vi "Main.vi"() -> ()   [LabVIEW 2021]
doc: "Use this template to build a simple state machine design pattern. Each state executes code and determines which state to transition to."
uses:
  controls/State.ctl
  controls/Data.ctl
  vmmso/vmmso.lvlib
panel:
  in  "DDS2 Amplitude":dbl=2000.0
  in  "DDS2 Bias":dbl
  in  "DDS2 Freq":dbl=1000.0
  in  "DDS2 Wave Style":u16(ring) items=["Sine", "Square", "Ramp"]
  in  "DDS1 Amplitude":dbl=2000.0
  in  "DDS1 Bias":dbl
  in  "DDS1 Freq":dbl=1000.0
  in  "DDS1 Wave Style":u16(ring) items=["Sine", "Square", "Ramp"]
  out "Is Data Ready？":bool
  out "ReadVoltageData Return":u32
  out "Voltage Wave":dbl[][](graph)
  out "Capture Return":i32
  out "Device is OK?":bool
  out "Support Samples":u32[](array[numeric])
  in  "Exit":bool
  # "DDS1"
  # "DDS2"
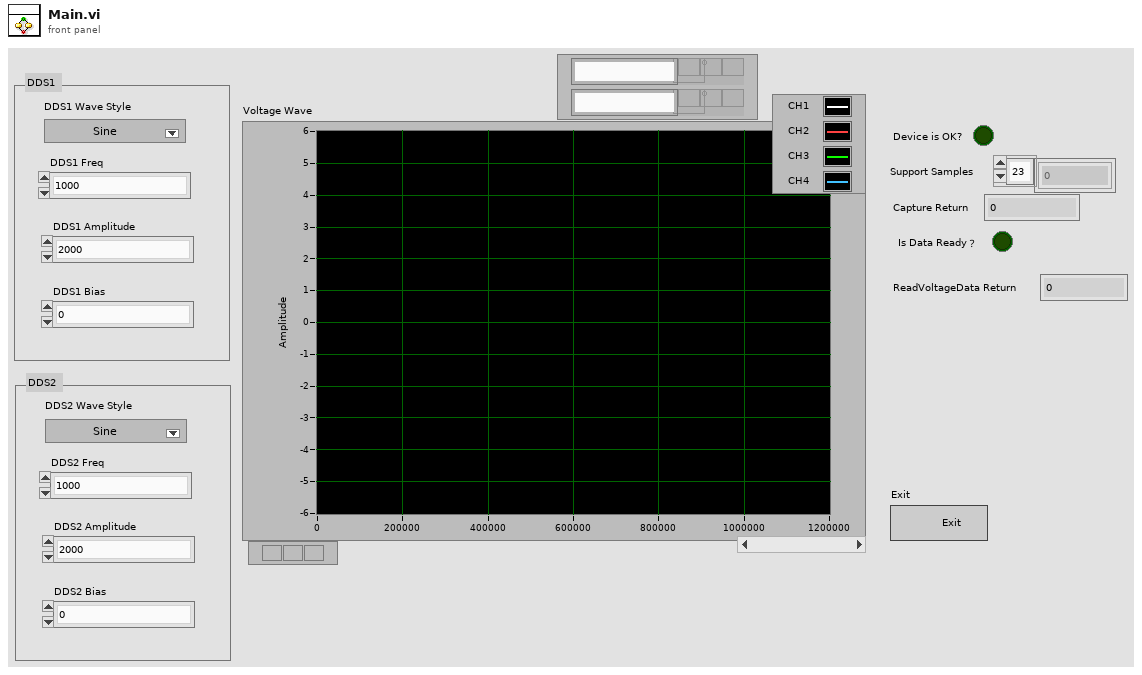
[diagram p1: front panel]
types:
  T1 = typedef "Data.ctl" = cluster{"Boolean <Replace Me>":bool, "String <Replace Me>":string, "Numeric <Replace Me>":dbl}
  T2 = typedef "State.ctl" = enum16{"Initialize", "Wait for UsbIn", "Init Osc and Dds", "Wait for Event", "Capture", "Read Voltage", "Exit"}
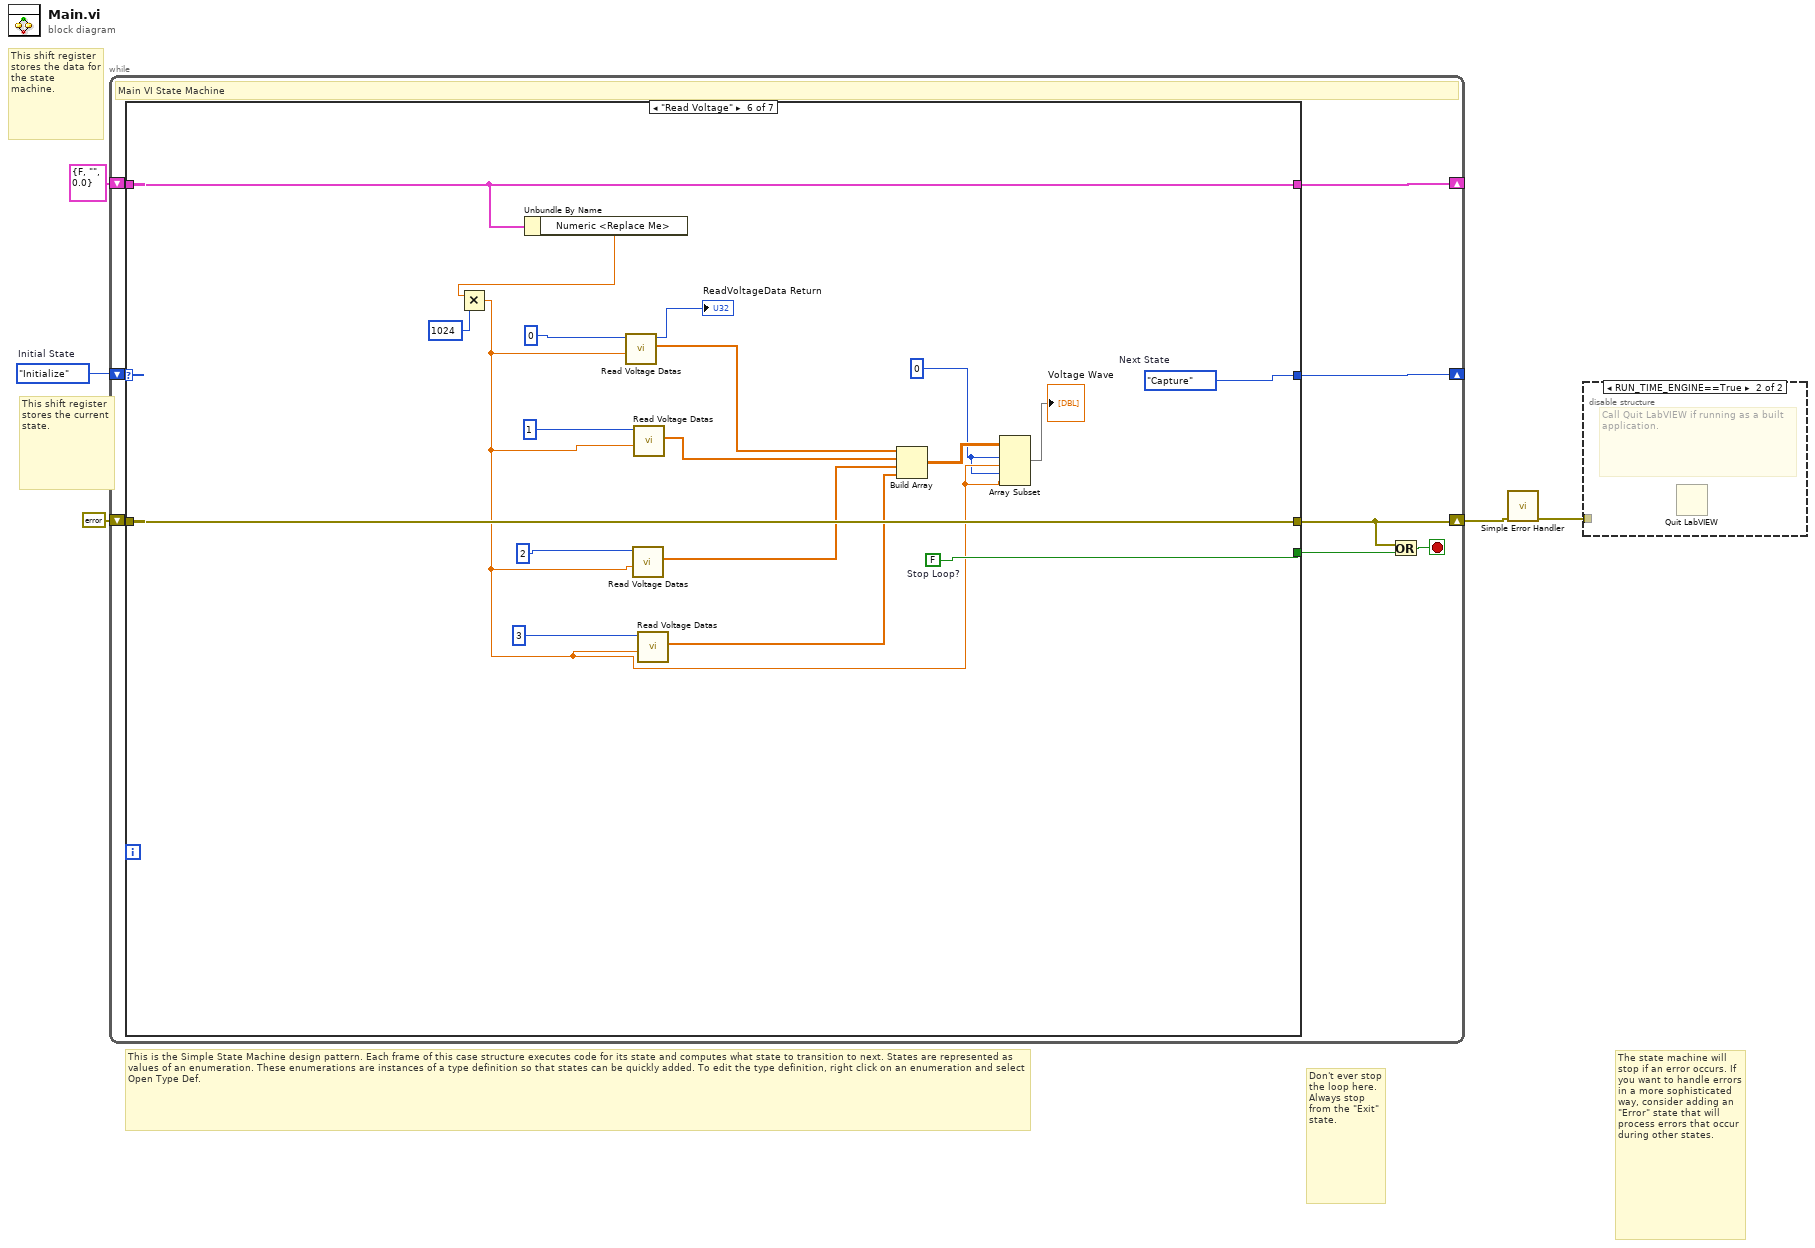
[diagram p0: block diagram]
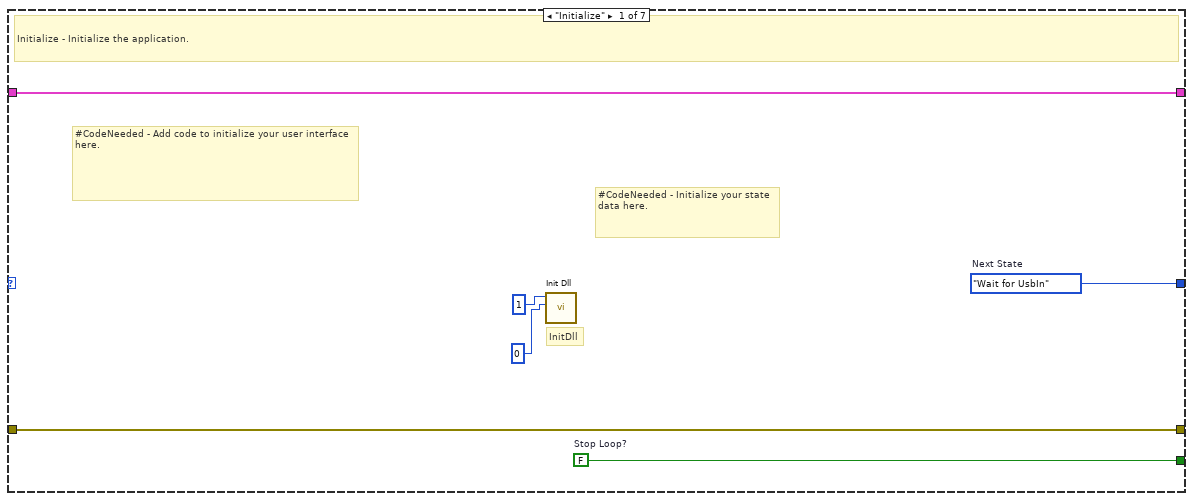
[diagram p3: hidden frame]
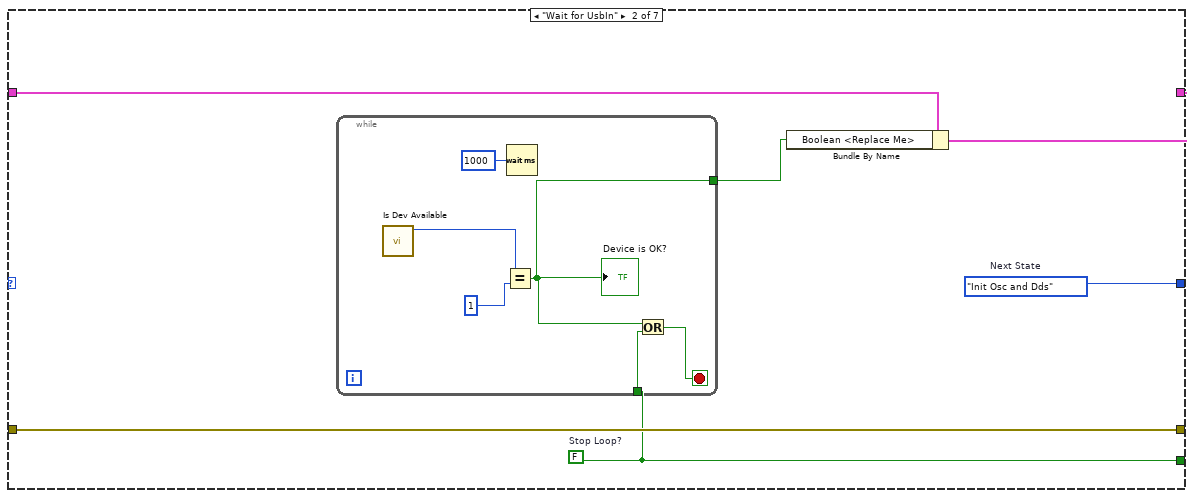
[diagram p4: hidden frame]
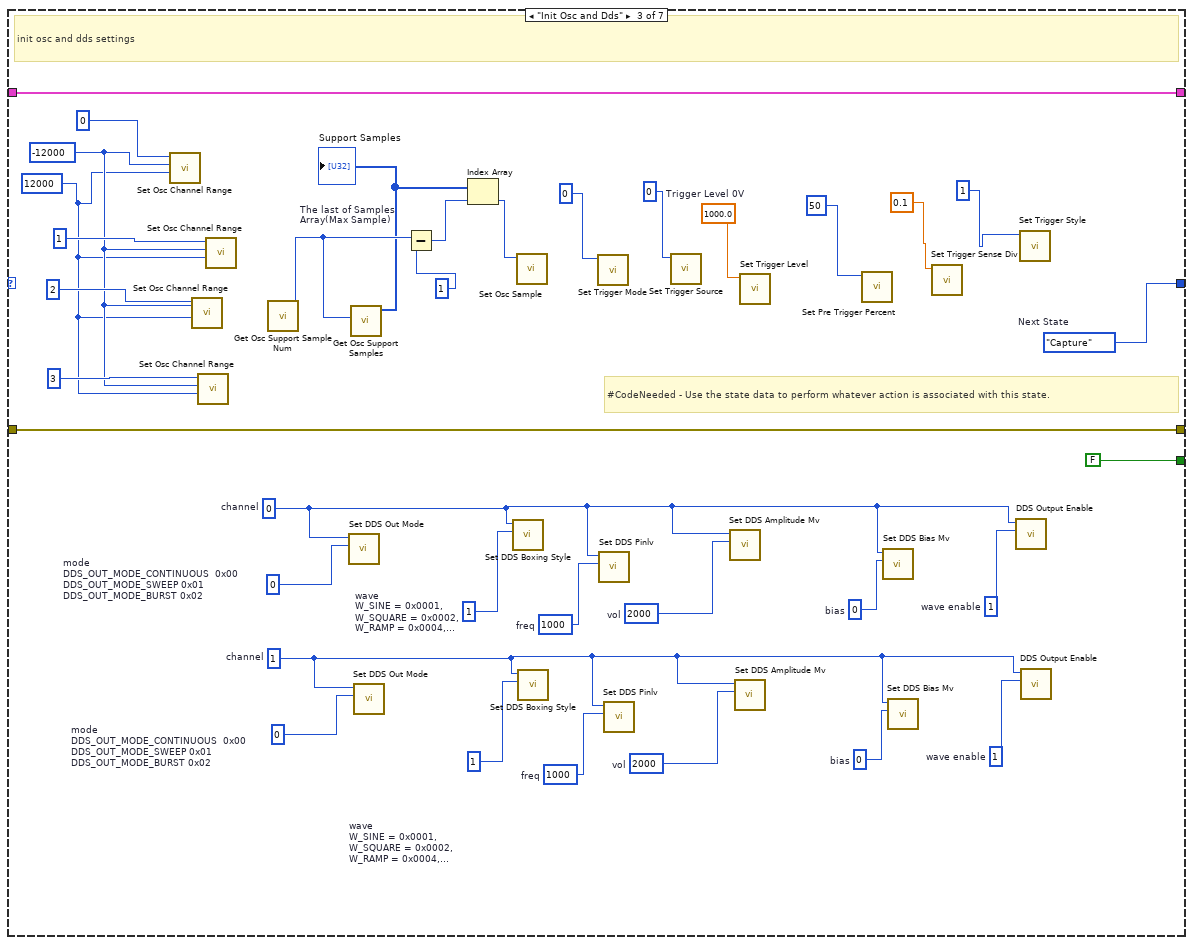
[diagram p5: hidden frame]
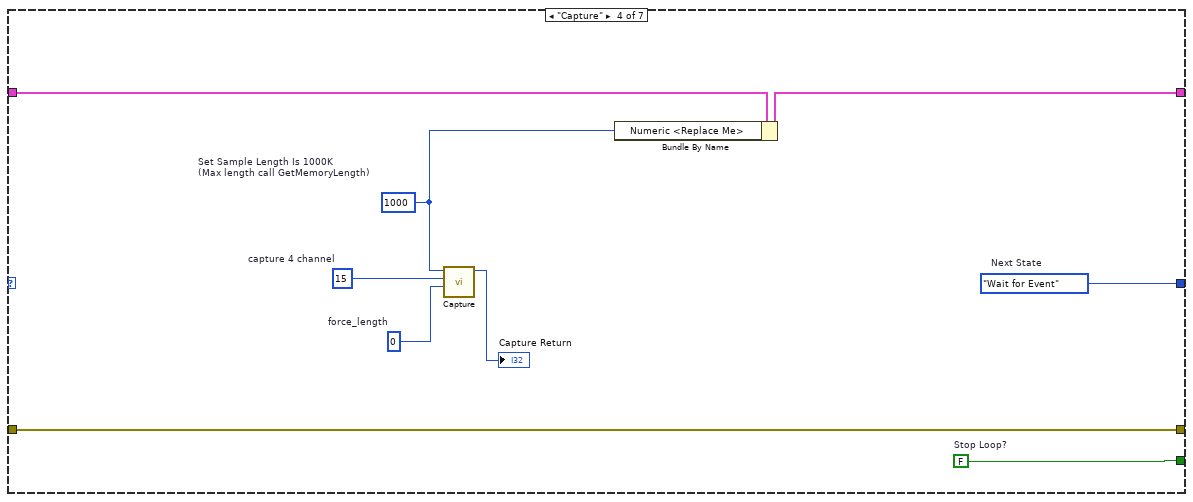
[diagram p6: hidden frame]
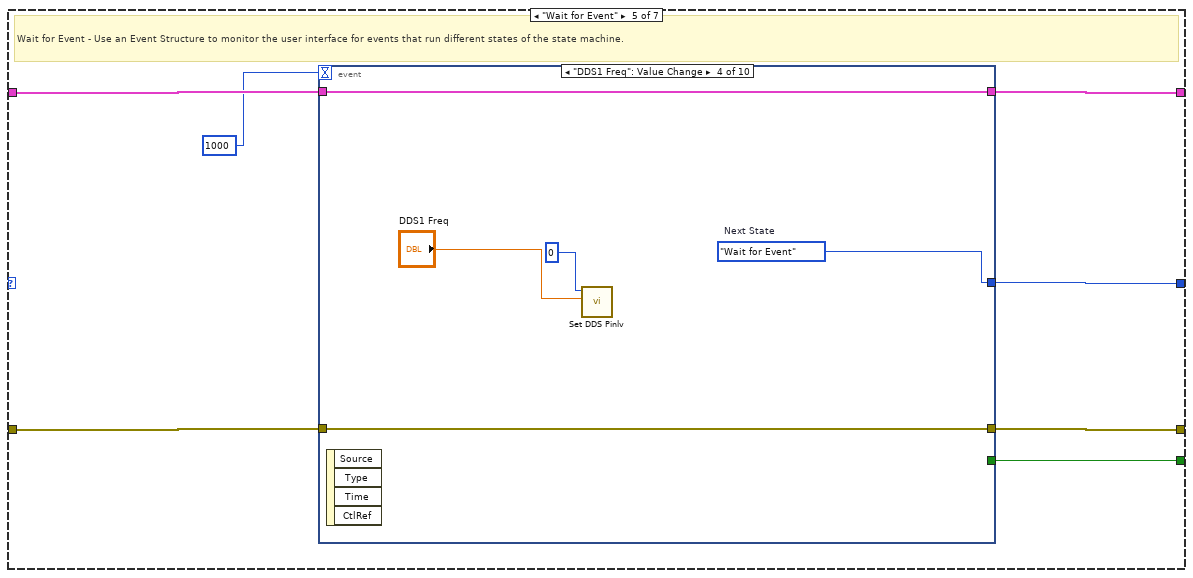
[diagram p7: hidden frame]
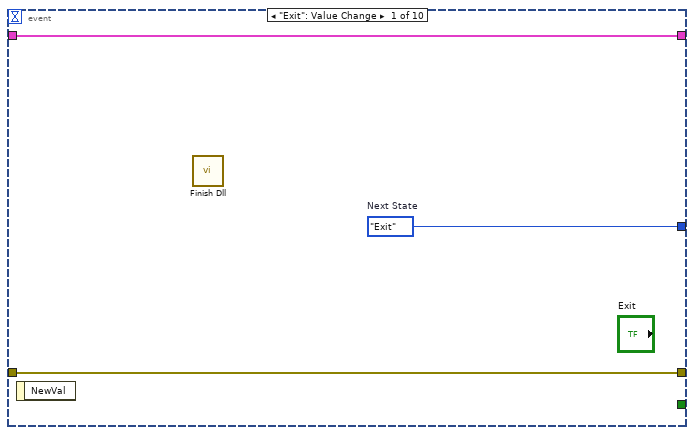
[diagram p8: hidden frame]
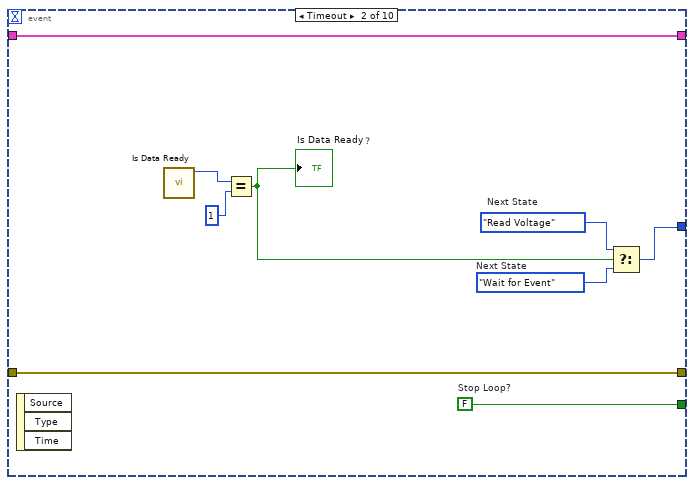
[diagram p9: hidden frame]
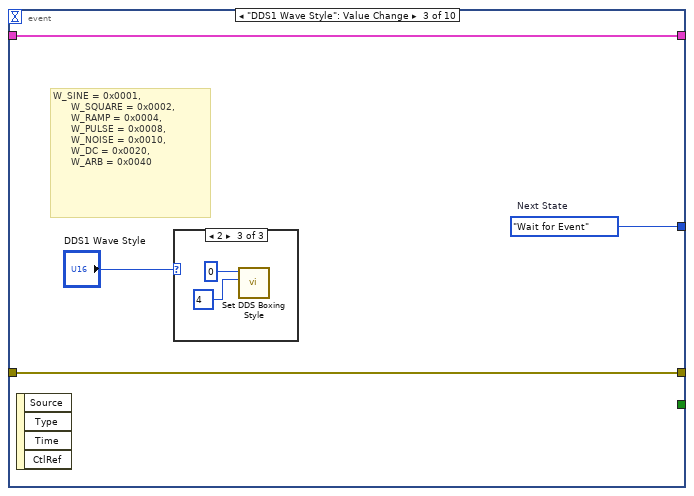
[diagram p10: hidden frame]
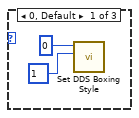
[diagram p11: hidden frame]
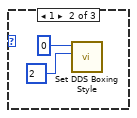
[diagram p12: hidden frame]
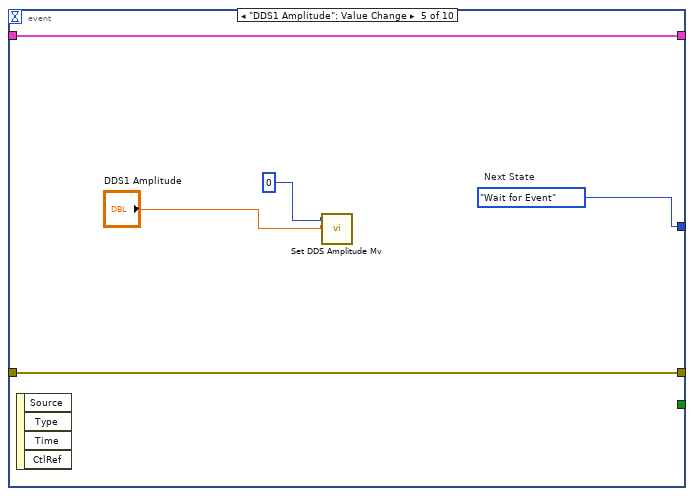
[diagram p13: hidden frame]
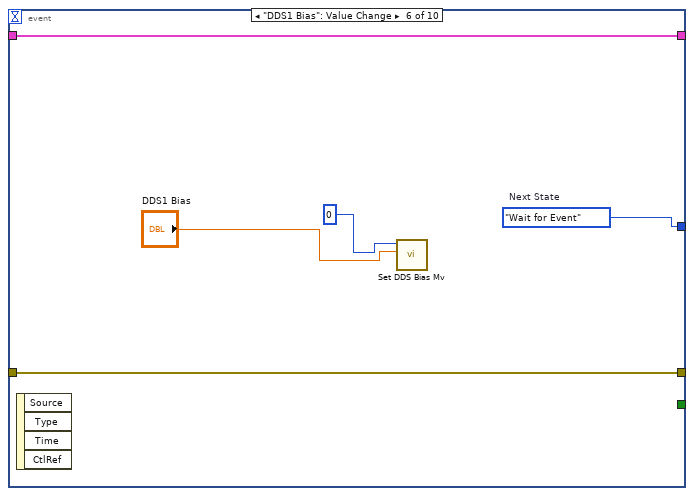
[diagram p14: hidden frame]
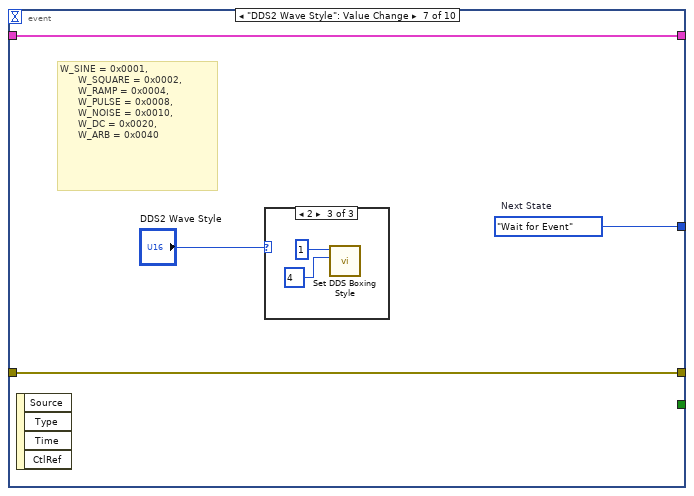
[diagram p15: hidden frame]
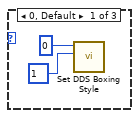
[diagram p16: hidden frame]
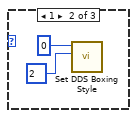
[diagram p17: hidden frame]
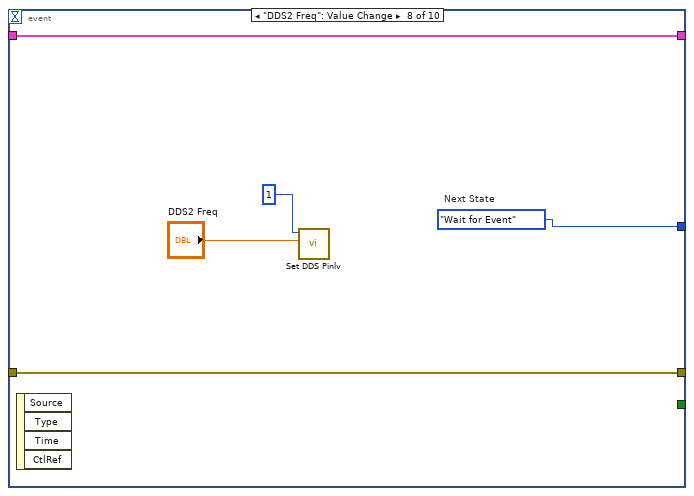
[diagram p18: hidden frame]
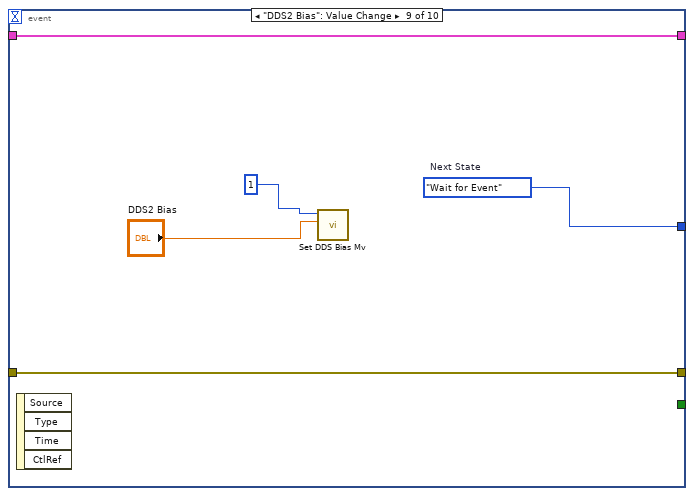
[diagram p19: hidden frame]
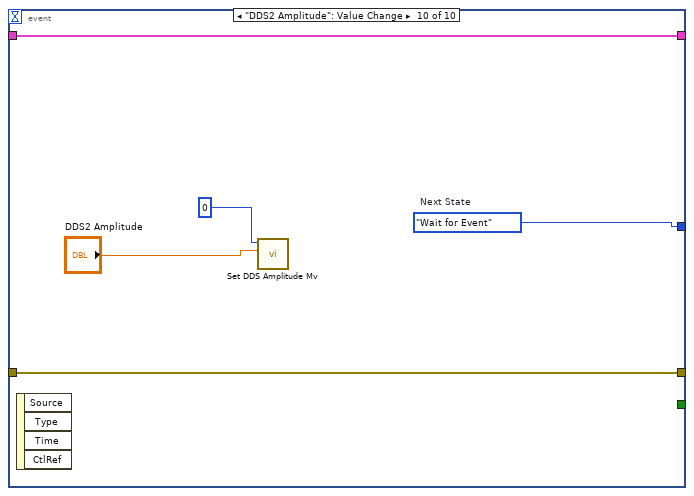
[diagram p20: hidden frame]
diagram:
  w5 = State."Initialize"  # Initial State
  # "Don't ever stop the loop here. Always stop from the \"Exit\" state."
  # "The state machine will stop if an error occurs. If you want to handle errors in a more sophisticated way, consider adding an \"Error\" state that will process errors that occur during other states."
  # "This shift register stores the data for the state machine."
  # "This is the Simple State Machine design pattern. Each frame of this case structure executes code for its state and computes what state to transition to next. States are represented as values of an enumeration. These enumerations are instances of a type definition so that states can be quickly added. To edit the type definition, right click on an enumeration and select Open Type Def."
  # "This shift register stores the current state."
  n1 = while {
    shift-right: [w12] -> _
    shift-left: w5 -> [w13]
    shift-right: [w10] -> _
    shift-left: T1 {"Boolean <Replace Me>"=FALSE, "String <Replace Me>"="", "Numeric <Replace Me>"=0.0} ("Data") -> [w11]
    shift-right: [w7] -> w2
    shift-left: errorcluster {"status"=FALSE, "code"=0, "source"=""} ("error constant") -> [w9]
    stop <- w8 stop-if-true
    # "Main VI State Machine"
    n2 = case shown="\"Read Voltage\"" w13 {
      tunnel: [w19 w24 w66 w74 w82 w161 w167] -> w12
      tunnel: w11 -> [w14 w22 w64 w69 w81 w157 w166]
      tunnel: [w14 w21 w64 w68 w80 w157 w166] -> w10
      tunnel: w9 -> [w17 w25 w63 w75 w79 w163 w164]
      tunnel: [w17 w25 w63 w75 w78 w163 w164] -> w7
      tunnel: [w18 w23 FALSE ("Stop Loop?") w73 w77 w162 w165] -> w6
      frame "Initialize" {
        w18 = FALSE  # Stop Loop?
        w19 = State."Wait for UsbIn"  # Next State
        # "InitDll"
        # "#CodeNeeded - Initialize your state data here."
        # "#CodeNeeded - Add code to initialize your user interface here."
        # "Initialize - Initialize the application."
        n3 = call "Init Dll.vi"("en_hard_watchdog"=0 ("channel"), "en_log"=1 ("channel")) -> ()  [unwired: 9 in, 1 out]
      }
      frame "Wait for UsbIn" {
        w24 = State."Init Osc and Dds"  # Next State
        w23 = FALSE  # Stop Loop?
        n4 = while {
          tunnel: w23 -> [w29]
          tunnel: [w26] -> w20
          stop <- w28 stop-if-true
          n5 = call "Is Dev Available.vi"() -> ("function return"=w27:i32)  [unwired: 11 in]
          n6 = Equal?(x=w27, y=1 ("channel")) -> (x = y?=w26:bool)
          "Device is OK?" <- w26
          n7 = Wait (ms)(milliseconds to wait=u32 1000 ("等待时间（毫秒）")) -> ()  [unwired: 1 out]
          n8 = Or(x=w26, y=w29) -> (x .or. y?=w28:bool)
        }
        n9 = Bundle By Name(cluster=w22, "Boolean <Replace Me>"=w20) -> (w21:T1)
      }
      frame "Init Osc and Dds" {
        w37 = i8 0  # mode DDS_OUT_MODE_CONTINUOUS  0x00 DDS_OUT_MODE_SWEEP 0x01 DDS_OUT_MODE_BURST 0x02
        w39 = i8 1  # wave enable
        w41 = u32 0  # bias
        w40 = u32 2000  # vol
        w42 = u32 1000  # freq
        w43 = i8 1  # wave  W_SINE = 0x0001,  W_SQUARE = 0x0002,  W_RAMP = 0x0004,  W_PULSE = 0x0008,  W_NOISE = 0x0010,  W_DC = 0x0020,  W_ARB = 0x0040
        w38 = i8 1  # channel
        w44 = i8 0  # mode DDS_OUT_MODE_CONTINUOUS  0x00 DDS_OUT_MODE_SWEEP 0x01 DDS_OUT_MODE_BURST 0x02
        w46 = i8 1  # wave enable
        w48 = u32 0  # bias
        w47 = u32 2000  # vol
        w49 = u32 1000  # freq
        w50 = i8 1  # wave  W_SINE = 0x0001,  W_SQUARE = 0x0002,  W_RAMP = 0x0004,  W_PULSE = 0x0008,  W_NOISE = 0x0010,  W_DC = 0x0020,  W_ARB = 0x0040
        w45 = i8 0  # channel
        w60 = sgl 1000.0  # Trigger Level 0V
        w32 = 12000 ("minmv")
        w33 = -12000 ("minmv")
        w66 = State."Capture"  # Next State
        # "#CodeNeeded - Use the state data to perform whatever action is associated with this state."
        # "init osc and dds settings"
        n10 = call "Set Osc Channel Range.vi"("maxmv"=w32, "minmv"=w33, "channel"=0) -> ()  [unwired: 8 in, 1 out]
        n11 = call "Set Osc Channel Range.vi"("maxmv"=w32, "minmv"=w33, "channel"=2) -> ()  [unwired: 8 in, 1 out]
        n12 = call "Set Osc Channel Range.vi"("maxmv"=w32, "minmv"=w33, "channel"=3) -> ()  [unwired: 8 in, 1 out]
        n13 = call "Set Osc Channel Range.vi"("maxmv"=w32, "minmv"=w33, "channel"=1) -> ()  [unwired: 8 in, 1 out]
        n14 = call "Get Osc Support Sample Num.vi"() -> ("function return"=w56:i32)  [unwired: 11 in]
        n15 = call "Set DDS Out Mode.vi"("out_mode"=w44, "channel_index"=w45) -> ()  [unwired: 10 in]
        n16 = call "Get Osc Support Samples.vi"("maxnum"=w56) -> ("sample out"=w53:u32[])  [unwired: 9 in, 1 out]
        "Support Samples" <- w53
        n17 = call "Set DDS Out Mode.vi"("out_mode"=w37, "channel_index"=w38) -> ()  [unwired: 10 in]
        n18 = Subtract "The last of Samples Array(Max Sample)"(x=w56, y=1 ("front")) -> (x-y=w58:i32)
        n19 = Index Array(array=w53, index=w58) -> (element=w59:u32)
        n20 = call "Set DDS Boxing Style.vi"("boxing"=w50, "channel_index"=w45) -> ()  [unwired: 10 in]
        n21 = call "Set Osc Sample.vi"("sample"=w59) -> ()  [unwired: 10 in, 1 out]
        n22 = call "Set DDS Boxing Style.vi"("boxing"=w43, "channel_index"=w38) -> ()  [unwired: 10 in]
        n23 = call "Set Trigger Mode.vi"("mode"=0 ("front")) -> ()  [unwired: 11 in]
        n24 = call "Set DDS Pinlv.vi"("pinlv"=w49, "channel_index"=w45) -> ()  [unwired: 10 in]
        n25 = call "Set DDS Pinlv.vi"("pinlv"=w42, "channel_index"=w38) -> ()  [unwired: 10 in]
        n26 = call "Set Trigger Source.vi"("source"=0 ("front")) -> ()  [unwired: 11 in]
        n27 = call "Set DDS Amplitude Mv.vi"("amplitdude"=w47, "channel_index"=w45) -> ()  [unwired: 10 in]
        n28 = call "Set DDS Amplitude Mv.vi"("amplitdude"=w40, "channel_index"=w38) -> ()  [unwired: 10 in]
        n29 = call "Set Trigger Level.vi"("level"=w60) -> ()  [unwired: 11 in]
        n30 = call "Set Pre Trigger Percent.vi"("front"=50) -> ()  [unwired: 11 in]
        n31 = call "Set DDS Bias Mv.vi"("bias"=w48, "channel_index"=w45) -> ()  [unwired: 10 in]
        n32 = call "Set DDS Bias Mv.vi"("bias"=w41, "channel_index"=w38) -> ()  [unwired: 10 in]
        n33 = call "Set Trigger Sense Div.vi"("sense"=0.1) -> ()  [unwired: 11 in]
        n34 = call "DDS Output Enable.vi"("enable"=w46, "channel_index"=w45) -> ()  [unwired: 10 in]
        n35 = call "Set Trigger Style.vi"("style"=u32 1) -> ()  [unwired: 11 in]
        n36 = call "DDS Output Enable.vi"("enable"=w39, "channel_index"=w38) -> ()  [unwired: 10 in]
      }
      frame "Capture" {
        w70 = i8 0  # force_length
        w67 = u32 1000  # Set Sample Length Is 1000K (Max length call GetMemoryLength)
        w71 = i8 15  # capture 4 channel
        w73 = FALSE  # Stop Loop?
        w74 = State."Wait for Event"  # Next State
        n37 = call "Capture.vi"("force_length"=w70, "capture_channel"=w71, "length"=w67) -> ("function return"=→"Capture Return":i32)  [unwired: 8 in]
        n38 = Bundle By Name(cluster=w69, "Numeric <Replace Me>"=w67) -> (w68:T1)
      }
      frame "Wait for Event" {
        # "Wait for Event - Use an Event Structure to monitor the user interface for events that run different states of the state machine."
        n39 = event shown="[3] \"DDS1 Freq\": Value Change" {
          selector: _ -> [_ _ _ _ _ _ _ _ _ _]
          dyn-events: _ -> [_ _ _ _ _ _ _ _ _ _]
          timeout: 1000 ("y") -> [_ _ _ _ _ _ _ _ _ _]
          tunnel: [w85 w89 w95 w107 w112 w117 w121 w131 w136 w141] -> w82
          tunnel: w81 -> [w84 w94 w98 w109 w114 w119 w123 w134 w139 w144]
          tunnel: [w84 w94 w98 w109 w114 w119 w123 w134 w139 w144] -> w80
          tunnel: w79 -> [w83 w93 w97 w108 w113 w118 w122 w133 w138 w143]
          tunnel: [w83 w93 w97 w108 w113 w118 w122 w133 w138 w143] -> w78
          tunnel: [_ w90 _ _ _ _ _ _ _ _] -> w77
          event "Exit": Value Change {
            w85 = State."Exit"  # Next State
            n40 = event-data() -> ()  [unwired: 1 in, 1 out]
            n41 = call "Finish Dll.vi"() -> ()  [unwired: 11 in, 1 out]
          }
          event Timeout {
            w86 = State."Wait for Event"  # Next State
            w90 = FALSE  # Stop Loop?
            w87 = State."Read Voltage"  # Next State
            n42 = event-data() -> ()  [unwired: 1 in, 3 out]
            n43 = call "Is Data Ready.vi"() -> ("function return"=w92:i32)  [unwired: 11 in]
            n44 = Equal?(x=w92, y=1) -> (x = y?=w88:bool)
            "Is Data Ready？" <- w88
            n45 = Select(t=w87, s=w88, f=w86) -> (s? t:f=w89:T2)
          }
          event "DDS1 Wave Style": Value Change {
            w95 = State."Wait for Event"  # Next State
            # "W_SINE = 0x0001, \n\t\t\t\t\t\tW_SQUARE = 0x0002, \n\t\t\t\t\t\tW_RAMP = 0x0004, \n\t\t\t\t\t\tW_PULSE = 0x0008, \n\t\t\t\t\t\tW_NOISE = 0x0010, \n\t\t\t\t\t\tW_DC = 0x0020, \n\t\t\t\t\t\tW_ARB = 0x0040"
            n46 = event-data() -> ()  [unwired: 1 in, 4 out]
            n47 = case shown="2" "DDS1 Wave Style" {
              frame 0, Default {
                n48 = call "Set DDS Boxing Style.vi"("boxing"=1 ("y"), "channel_index"=0 ("y")) -> ()  [unwired: 10 in]
              }
              frame 1 {
                n49 = call "Set DDS Boxing Style.vi"("boxing"=2 ("y"), "channel_index"=0 ("y")) -> ()  [unwired: 10 in]
              }
              frame 2 {
                n50 = call "Set DDS Boxing Style.vi"("boxing"=4 ("y"), "channel_index"=0 ("y")) -> ()  [unwired: 10 in]
              }
            }
          }
          event "DDS1 Freq": Value Change {
            w107 = State."Wait for Event"  # Next State
            n51 = event-data() -> ()  [unwired: 1 in, 4 out]
            n52 = call "Set DDS Pinlv.vi"("pinlv"="DDS1 Freq", "channel_index"=0 ("y")) -> ()  [unwired: 10 in]
          }
          event "DDS1 Amplitude": Value Change {
            w112 = State."Wait for Event"  # Next State
            n53 = event-data() -> ()  [unwired: 1 in, 4 out]
            n54 = call "Set DDS Amplitude Mv.vi"("amplitdude"="DDS1 Amplitude", "channel_index"=0 ("y")) -> ()  [unwired: 10 in]
          }
          event "DDS1 Bias": Value Change {
            w117 = State."Wait for Event"  # Next State
            n55 = event-data() -> ()  [unwired: 1 in, 4 out]
            n56 = call "Set DDS Bias Mv.vi"("bias"="DDS1 Bias", "channel_index"=0 ("y")) -> ()  [unwired: 10 in]
          }
          event "DDS2 Wave Style": Value Change {
            w121 = State."Wait for Event"  # Next State
            # "W_SINE = 0x0001, \n\t\t\t\t\t\tW_SQUARE = 0x0002, \n\t\t\t\t\t\tW_RAMP = 0x0004, \n\t\t\t\t\t\tW_PULSE = 0x0008, \n\t\t\t\t\t\tW_NOISE = 0x0010, \n\t\t\t\t\t\tW_DC = 0x0020, \n\t\t\t\t\t\tW_ARB = 0x0040"
            n57 = event-data() -> ()  [unwired: 1 in, 4 out]
            n58 = case shown="2" "DDS2 Wave Style" {
              frame 0, Default {
                n59 = call "Set DDS Boxing Style.vi"("boxing"=1 ("y"), "channel_index"=0 ("y")) -> ()  [unwired: 10 in]
              }
              frame 1 {
                n60 = call "Set DDS Boxing Style.vi"("boxing"=2 ("y"), "channel_index"=0 ("y")) -> ()  [unwired: 10 in]
              }
              frame 2 {
                n61 = call "Set DDS Boxing Style.vi"("boxing"=4 ("y"), "channel_index"=1 ("y")) -> ()  [unwired: 10 in]
              }
            }
          }
          event "DDS2 Freq": Value Change {
            w131 = State."Wait for Event"  # Next State
            n62 = event-data() -> ()  [unwired: 1 in, 4 out]
            n63 = call "Set DDS Pinlv.vi"("pinlv"="DDS2 Freq", "channel_index"=1 ("y")) -> ()  [unwired: 10 in]
          }
          event "DDS2 Bias": Value Change {
            w136 = State."Wait for Event"  # Next State
            n64 = event-data() -> ()  [unwired: 1 in, 4 out]
            n65 = call "Set DDS Bias Mv.vi"("bias"="DDS2 Bias", "channel_index"=1 ("y")) -> ()  [unwired: 10 in]
          }
          event "DDS2 Amplitude": Value Change {
            w141 = State."Wait for Event"  # Next State
            n66 = event-data() -> ()  [unwired: 1 in, 4 out]
            n67 = call "Set DDS Amplitude Mv.vi"("amplitdude"="DDS2 Amplitude", "channel_index"=0 ("y")) -> ()  [unwired: 10 in]
          }
        }
      }
      frame "Read Voltage" {
        w147 = i8 0 ("channel")
        w161 = State."Capture"  # Next State
        w162 = FALSE  # Stop Loop?
        n68 = Unbundle By Name(w157) -> ("Numeric <Replace Me>"=w156:dbl)
        n69 = Multiply(x=w156, y=1024) -> (x*y=w148:dbl)
        n70 = call "Read Voltage Datas.vi"("length"=w148, "channel"=i8 0) -> ("buffer out"=w145:dbl[], "function return"=→"ReadVoltageData Return":u32)  [unwired: 8 in]
        n71 = call "Read Voltage Datas.vi"("length"=w148, "channel"=i8 2) -> ("buffer out"=w151:dbl[])  [unwired: 8 in, 1 out]
        n72 = call "Read Voltage Datas.vi"("length"=w148, "channel"=i8 1) -> ("buffer out"=w152:dbl[])  [unwired: 8 in, 1 out]
        n73 = call "Read Voltage Datas.vi"("length"=w148, "channel"=i8 3) -> ("buffer out"=w150:dbl[])  [unwired: 8 in, 1 out]
        n74 = Build Array(w145, w152, w151, w150) -> (w149:dbl[][])
        n75 = Array Subset(array=w149, index (row)=w147, length (row)=w148, index (col)=w147, length (col)=w148) -> (→"Voltage Wave":dbl[][])
      }
      frame "Exit" {
        w165 = TRUE  # Stop Loop?
        w167 = State."Exit"  # (Value Not Used)
        # "#CodeNeeded - Add any required cleanup code here."
        # "The state value is not used here since this is the last iteration of the state machine loop."
        # "Exit - Exit the application."
      }
    }
    n76 = Or(x=w7, y=w6) -> (x .or. y?=w8:bool)
  }
  n77 = call <vilib>:"Simple Error Handler.vi"("error in (no error)"=w2) -> ("error out"=w1:errorcluster)  [unwired: 4 in, 4 out]
  n78 = disable-structure shown="RUN_TIME_ENGINE==True" {
    disable-tunnel: w1 -> [_ _]
    frame condition #0 (active) {
    }
    frame condition #1 {
      # "Call Quit LabVIEW if running as a built application."
      n79 = Quit LabVIEW() -> ()  [unwired: 1 in]
    }
  }
